vi "Mean Range Values from FP Indicators.vi"(8 "error in (no error)":errorcluster, 11 "MWWL Verification in":refnum<class "MWWL Verification.lvclass">) -> (0 "error out":errorcluster, 2 "Mean Range Value":dbl, 3 "MWWL Verification out":refnum<class "MWWL Verification.lvclass">)   [LabVIEW 2018, in "MWWL Verification.lvlib" / "MWWL Verification.lvclass"]
uses:
  MWWL Verification.lvclass
  MWWL Verification.lvclass/MWWL Verification.ctl
  <vilib>/gmath/NI_Gmath.lvlib
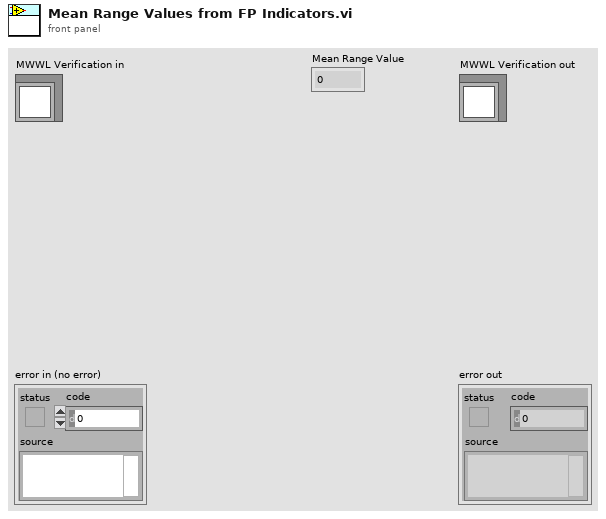
[diagram p1: front panel]
types:
  T1 = cluster{"ULS A":bool, "ULS B":bool, "ULS C":bool, "ULS D":bool}
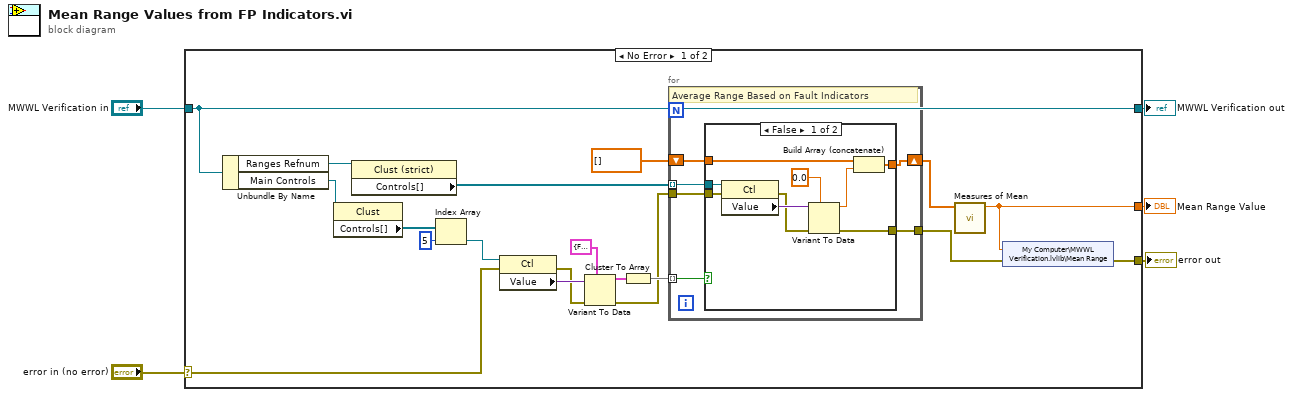
[diagram p0: block diagram]
diagram:
  n1 = case shown="No Error" "error in (no error)" {
    selector: "error in (no error)" -> [w13 w43]
    tunnel: [w18 w43] -> w4
    tunnel: [w24 w42] -> w2
    tunnel: "MWWL Verification in" -> [w24 w42]
    tunnel: [w22 _] -> w1
    frame No Error {
      n2 = Unbundle By Name(w24) -> ("Ranges Refnum"=w23:refnum<vi>, "Main Controls"=w20:refnum<vi>)
      n3 = property class="Clust"(reference=w20) -> ("Controls[]"=w17:refnum<vi>[])  [unwired: 1 in, 2 out]
      n4 = property class="Clust (strict)"(reference=w23) -> ("Controls[]"=w21:refnum<vi>[])  [unwired: 1 in, 2 out]
      n5 = Index Array(array=w17, index=5) -> (element=w15:refnum<vi>)
      n6 = property class="Ctl"(reference=w15, error in=w13) -> (error out=w12:errorcluster, "Value"=w14:variant)  [unwired: 1 out]
      n7 = Variant To Data(error in=w12, type=T1 {"ULS A"=FALSE, "ULS B"=FALSE, "ULS C"=FALSE, "ULS D"=FALSE} ("ULS Status"), Variant=w14) -> (data=w10:T1, error out=w6:errorcluster)
      n8 = Cluster To Array(cluster=w10) -> (array=w9:bool[])
      n9 = for {
        tunnel: w21 -> [w30] mode=indexing
        tunnel: w6 -> [w29]
        tunnel: [w26] -> w19
        tunnel: w9 -> [w25] mode=indexing
        shift-right: [w28] -> w7
        shift-left: dbl[] [] -> [w27]
        # "Average Range Based on Fault Indicators"
        n10 = case shown="False" w25 {
          tunnel: w30 -> [w39 _]
          tunnel: w29 -> [w36 w41]
          tunnel: [w34 w40] -> w28
          tunnel: w27 -> [w33 w40]
          tunnel: [w31 w41] -> w26
          frame False {
            n11 = property class="Ctl"(reference=w39, error in=w36) -> (error out=w35:errorcluster, "Value"=w38:variant)  [unwired: 1 out]
            n12 = Variant To Data(error in=w35, type=0.0, Variant=w38) -> (data=w32:dbl, error out=w31:errorcluster)
            n13 = Build Array (concatenate)(w33, w32) -> (w34:dbl[])
          }
          frame True {
          }
        }
      }
      n14 = call <vilib>:"Measures of Mean.vi"("x array"=w7) -> ("mean value"=w22:dbl)  [unwired: 9 in, 1 out]
      n15 = shared-variable "My Computer\\MWWL Verification.lvlib\\Mean Range"(w22, error in=w19) -> (error out=w18:errorcluster)
    }
    frame Error {
    }
  }
  "error out" <- w4
  "MWWL Verification out" <- w2
  "Mean Range Value" <- w1
